vi "aptmotorcontrol_Aaron_Edit.vi"() -> ()   [LabVIEW 2013]
panel:
  in  "Numeric":dbl
  out "pfPosition 3":sgl
  out "pfPosition 2":sgl
  in  "Serial 3":i32=90848556
  in  "MG17Motor 3":refnum<k7>(container)
  in  "Serial 2":i32=90848555
  in  "MG17Motor 2":refnum<k7>(container)
  out "pfPosition":sgl
  in  "MG17Motor":refnum<k7>(container)
  in  "stop":bool
  in  "Serial":i32=90848557
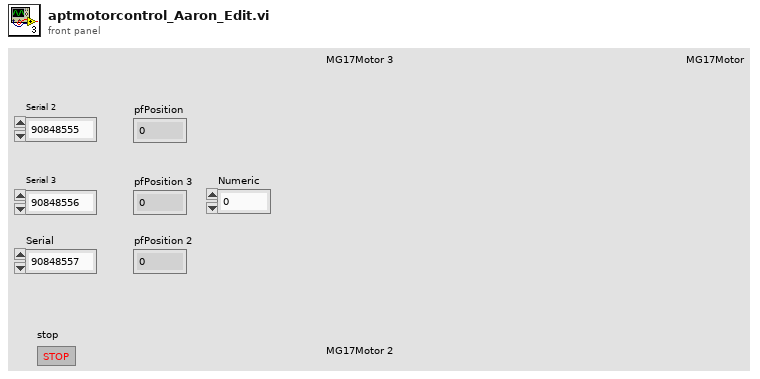
[diagram p1: front panel]
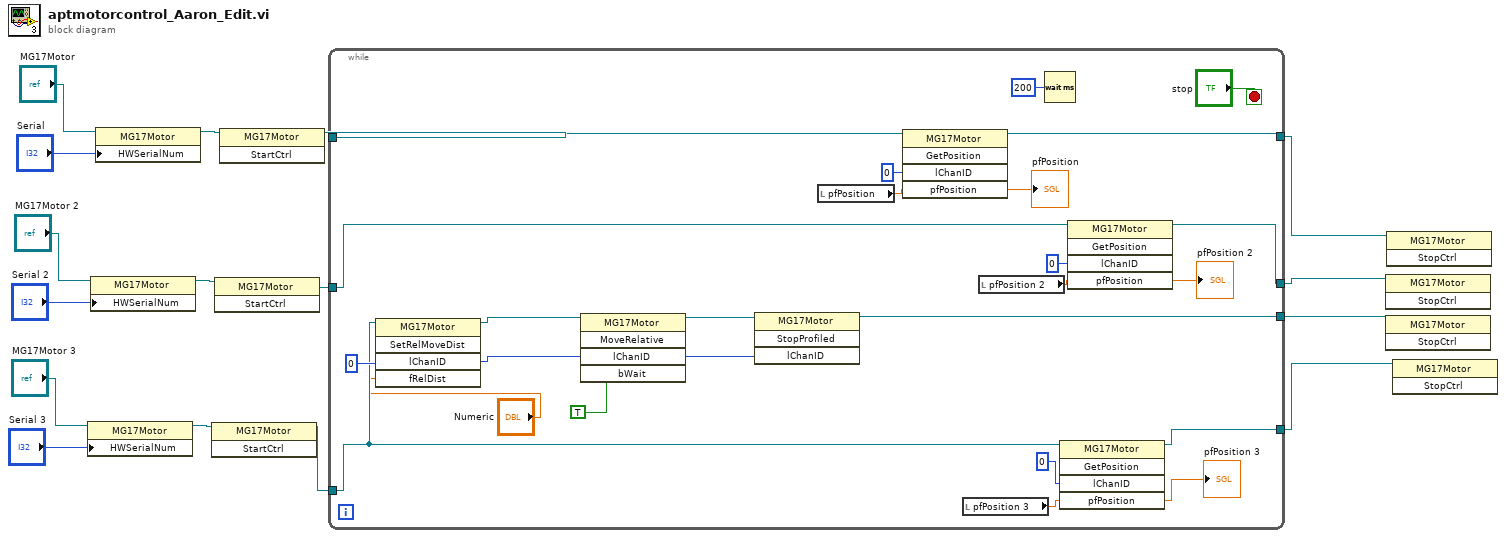
[diagram p0: block diagram]
diagram:
  n1 = property class="MG17Motor"(reference="MG17Motor 3", "HWSerialNum"="Serial 3") -> (reference out=w6:refnum<k7>)  [unwired: 1 in, 1 out]
  n2 = property class="MG17Motor"(reference="MG17Motor 2", "HWSerialNum"="Serial 2") -> (reference out=w9:refnum<k7>)  [unwired: 1 in, 1 out]
  n3 = property class="MG17Motor"(reference="MG17Motor", "HWSerialNum"="Serial") -> (reference out=w12:refnum<k7>)  [unwired: 1 in, 1 out]
  n4 = invoke class="MG17Motor" method="StartCtrl"(reference=w6) -> (reference out=w3:refnum<k7>)  [unwired: 2 in, 2 out]
  n5 = invoke class="MG17Motor" method="StartCtrl"(reference=w9) -> (reference out=w5:refnum<k7>)  [unwired: 2 in, 2 out]
  n6 = invoke class="MG17Motor" method="StartCtrl"(reference=w12) -> (reference out=w14:refnum<k7>)  [unwired: 2 in, 2 out]
  n7 = while {
    tunnel: w14 -> [w40]
    tunnel: [w39] -> w13
    tunnel: w5 -> [w31]
    tunnel: [w30] -> w4
    tunnel: w3 -> [w24]
    tunnel: [w26] -> w2
    tunnel: [w18] -> w1
    stop <- "stop" stop-if-true
    n8 = invoke class="MG17Motor" method="SetRelMoveDist"(reference=w24, "lChanID"=0, "fRelDist"="Numeric") -> (reference out=w22:refnum<k7>, "lChanID"=w21:i32)  [unwired: 2 in, 3 out]
    n9 = invoke class="MG17Motor" method="MoveRelative"(reference=w22, "lChanID"=w21, "bWait"=TRUE) -> (reference out=w20:refnum<k7>, "lChanID"=w19:i32)  [unwired: 2 in, 3 out]
    n10 = invoke class="MG17Motor" method="StopProfiled"(reference=w20, "lChanID"=w19) -> (reference out=w18:refnum<k7>)  [unwired: 2 in, 3 out]
    n11 = local read "pfPosition"() -> (w36:sgl)
    n12 = invoke class="MG17Motor" method="GetPosition"(reference=w40, "lChanID"=0, "pfPosition"=w36) -> (reference out=w39:refnum<k7>, "pfPosition"=→"pfPosition":sgl)  [unwired: 2 in, 3 out]
    n13 = local read "pfPosition 3"() -> (w27:sgl)
    n14 = local read "pfPosition 2"() -> (w34:sgl)
    n15 = Wait (ms)(milliseconds to wait=u32 200) -> ()  [unwired: 1 out]
    n16 = invoke class="MG17Motor" method="GetPosition"(reference=w24, "lChanID"=0, "pfPosition"=w27) -> (reference out=w26:refnum<k7>, "pfPosition"=→"pfPosition 3":sgl)  [unwired: 2 in, 3 out]
    n17 = invoke class="MG17Motor" method="GetPosition"(reference=w31, "lChanID"=0, "pfPosition"=w34) -> (reference out=w30:refnum<k7>, "pfPosition"=→"pfPosition 2":sgl)  [unwired: 2 in, 3 out]
  }
  n18 = invoke class="MG17Motor" method="StopCtrl"(reference=w4) -> ()  [unwired: 2 in, 3 out]
  n19 = invoke class="MG17Motor" method="StopCtrl"(reference=w1) -> ()  [unwired: 2 in, 3 out]
  n20 = invoke class="MG17Motor" method="StopCtrl"(reference=w13) -> ()  [unwired: 2 in, 3 out]
  n21 = invoke class="MG17Motor" method="StopCtrl"(reference=w2) -> ()  [unwired: 2 in, 3 out]
